vi "sv_Set Top and Bottom for MSG Plot Areas.vi"(9 "vertical margins":T1={"top offset"=20, "vertical space"=10, "bottom offset"=49}, 10 "height percentages":cluster{i32[]}[](array[cluster])=[{[50, 50]}, {[50, 50]}, {[50, 50]}, {[50, 50]}, {[20, 50, 30]}], 11 "references":refnum<vi>[](array[refnum])) -> ()   [LabVIEW 2017]
doc: "This subVI sets the plot heights on all Mixed Signal Graphs (MSGs) in array of input <b>references</b> according to the specified vertical margins and height percentages. This subVI functionality and default values were specifically developed for the Advanced Impact Test Example."
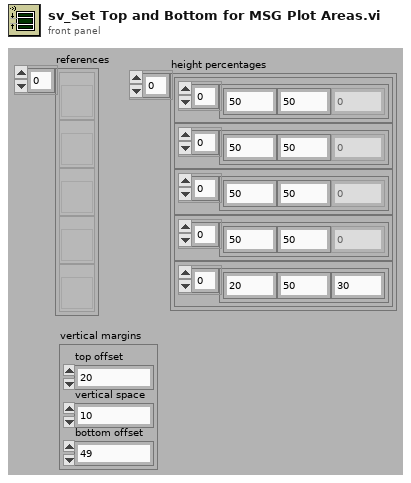
[diagram p1: front panel]
types:
  T1 = cluster{"top offset":i16, "vertical space":i16, "bottom offset":i16}
  T2 = typedef "LVRectTypeDef.ctl" = cluster{"Left":i16, "Top":i16, "Right":i16, "Bottom":i16}
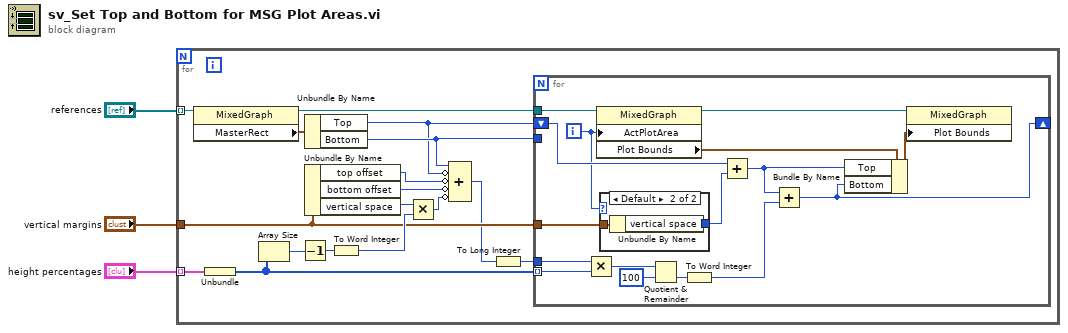
[diagram p0: block diagram]
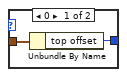
[diagram p2: hidden frame]
diagram:
  n1 = for {
    tunnel: "references" -> [w16] mode=indexing
    tunnel: "vertical margins" -> [w6]
    tunnel: "height percentages" -> [w20] mode=indexing
    n2 = property class="MixedGraph"(reference=w16) -> (reference out=w15:refnum<vi>, "MasterRect"=w14:T2)  [unwired: 1 in, 1 out]
    n3 = Unbundle(w20) -> (w19:i32[])
    n4 = Array Size(array=w19) -> (size(s)=w18:i32)
    n5 = Decrement(x=w18) -> (x-1=w17:i32)
    n6 = Unbundle By Name(w14) -> ("Top"=w8:i16, "Bottom"=w9:i16)
    n7 = Unbundle By Name(w6) -> ("top offset"=w11:i16, "bottom offset"=w12:i16, "vertical space"=w10:i16)
    n8 = To Word Integer(number=w17) -> (16bit integer=w7:i16)
    n9 = Multiply(x=w10, y=w7) -> (x*y=w13:i16)
    n10 = Compound Arithmetic op=ADD(w9, invert w8, invert w11, invert w12, invert w13) -> (w5:i16)
    n11 = To Long Integer(number=w5) -> (32bit integer=w4:i32)
    n12 = for {
      tunnel: w15 -> [w36]
      tunnel: w6 -> [w32]
      tunnel: w19 -> [w29] mode=indexing
      tunnel: w9 -> [_]
      shift-right: [w21] -> _
      shift-left: w8 -> [w30]
      tunnel: w4 -> [w25]
      i -> [w24]
      n13 = Multiply(x=w25, y=w29) -> (x*y=w28:i32)
      n14 = property class="MixedGraph"(reference=w36, "ActPlotArea"=w24) -> (reference out=w35:refnum<vi>, "Plot Bounds"=w34:T2)  [unwired: 1 in, 1 out]
      n15 = case shown="Default" w24 {
        tunnel: w32 -> [w38 w40]
        tunnel: [w37 w39] -> w31
        frame 0 {
          n16 = Unbundle By Name(w38) -> ("top offset"=w37:i16)
        }
        frame Default {
          n17 = Unbundle By Name(w40) -> ("vertical space"=w39:i16)
        }
      }
      n18 = Quotient & Remainder(x=w28, y=100) -> (floor(x/y)=w26:i32)  [unwired: 1 out]
      n19 = To Word Integer(number=w26) -> (16bit integer=w22:i16)
      n20 = Add(x=w30, y=w31) -> (x+y=w23:i16)
      n21 = Add(x=w23, y=w22) -> (x+y=w21:i16)
      n22 = Bundle By Name(cluster=w34, "Top"=w23, "Bottom"=w21) -> (w33:T2)
      n23 = property class="MixedGraph"(reference=w35, "Plot Bounds"=w33) -> ()  [unwired: 1 in, 2 out]
    }
  }
